vi "ParseURI.vi"(8 "error in":errorcluster, 11 "URI":string) -> (0 "error out":errorcluster, 1 "path":string, 2 "authority":string, 3 "scheme":string, 4 "query":string, 6 "fragment":string)   [LabVIEW 2013, in "openURI.lvlib"]
uses:
  openURI.lvlib
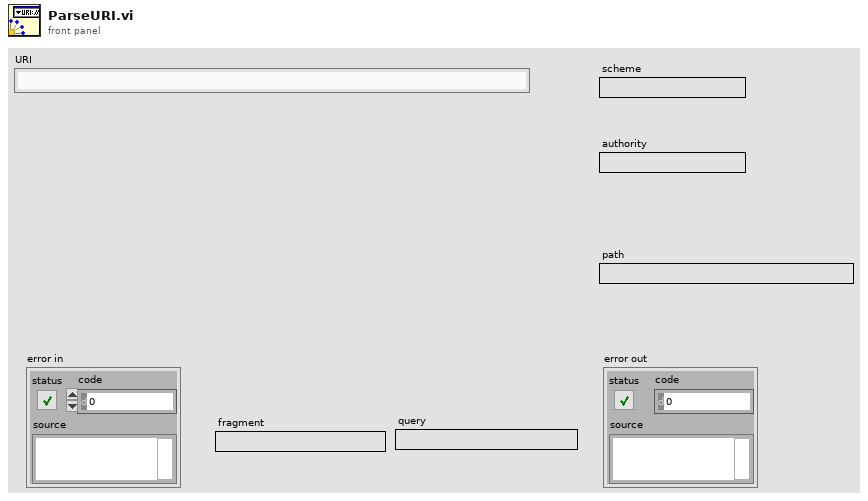
[diagram p1: front panel]
types:
  T1 = typedef "openURI.lvlib/URI Components -- cluster.ctl" = cluster{"scheme":string, "authority":string, "path":string, "query":string, "fragment":string}
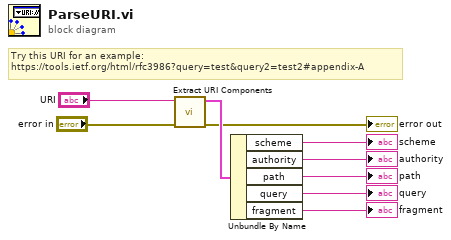
[diagram p0: block diagram]
diagram:
  # "Try this URI for an example:\nhttps://tools.ietf.org/html/rfc3986?query=test&query2=test2#appendix-A"
  n1 = call "Extract URI Components.vi"("error in"="error in", "URI"="URI") -> ("error out"=→"error out":errorcluster, "URI Components"=w8:T1)  [unwired: 8 in]
  n2 = Unbundle By Name(w8) -> ("scheme"=→"scheme":string, "authority"=→"authority":string, "path"=→"path":string, "query"=→"query":string, "fragment"=→"fragment":string)
